vi "TracepointDeviceResources.vi"(8 "error in (no error)":errorcluster, 9 "Mem":dbl format="%#_13g", 10 "CPU":dbl format="%#_13g", 11 "Qbus":refnum<class "Qbus.lvclass">) -> (0 "error out":errorcluster)   [LabVIEW 2017, in "DataAccumulator.lvlib"]
uses:
  <vilib>/addons/InsightCM/Devices/Shared/Common/DataAccumulator/DataAccumulator.lvlib
  <vilib>/addons/Qbus/Qbus.lvclass
  <vilib>/addons/TraceLogger/TraceLogger.lvlib
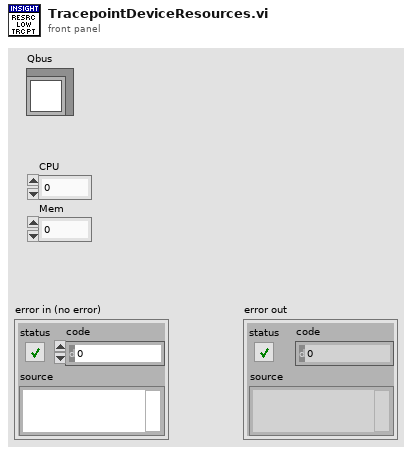
[diagram p1: front panel]
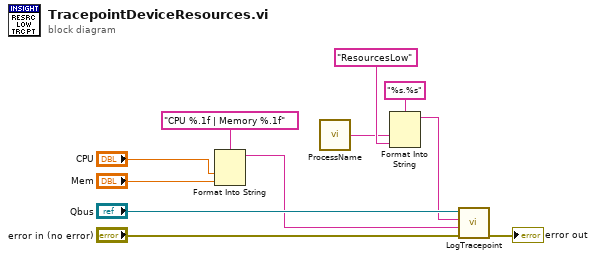
[diagram p0: block diagram]
diagram:
  n1 = Format Into String(format string="CPU %.1f | Memory %.1f", "CPU", "Mem") -> (resulting string=w1:string)  [unwired: 2 in, 1 out]
  n2 = call <vilib>:"ProcessName.vi"() -> ("process name"=w7:string)  [unwired: 5 in]
  n3 = Format Into String(format string="%s.%s", w7, "ResourcesLow" ("tracepoint")) -> (resulting string=w8:string)  [unwired: 2 in, 1 out]
  n4 = call <vilib>:"LogTracepoint.vi"("error in (no error)"="error in (no error)", "log string"=w1, "tracepoint"=w8, "qbus in"="Qbus") -> ("error out"=→"error out":errorcluster)  [unwired: 6 in, 1 out]
